vi "Mask Image to ROIs.vi"(8 "Error In":errorcluster, 9 "Max number of vectors in ROI (2500)":i32=2500, 10 "External edges only (T)":bool=TRUE, 11 "Mask Image Refnum in":T2) -> (0 "Error Out":errorcluster, 2 "ROIs":T1[](array[typedef]) {"Contours"."Type" items=["No Selection", "Point", "Line", "Rectangle", "Oval", "Polygon", "Freehand Region", "Annulus", "Unused2", "Unused3", "Broken Line", "Freehand Line", "Rotated Rectangle"]}, 3 "Mask Image Refnum out":T2)   [LabVIEW 2021, in "Image.lvlib"]
uses:
  <vilib>/vision/Image Controls.llb/IMAQ Image.ctl
  <userlib>/_OpenG.lib/array/array.llb/Filter 1D Array with Scalar (I32)__ogtk.vi
  Image.lvlib
  <vilib>/vision/NI_Vision_Development_Module.lvlib
  <userlib>/_OpenG.lib/array/array.llb/openg_array.lvlib
panel:
  out "# ROIs":i32
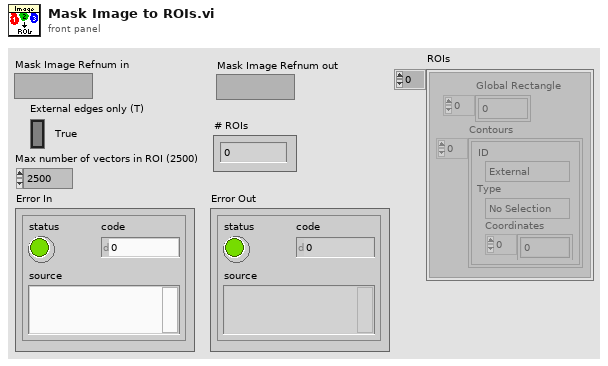
[diagram p1: front panel]
types:
  T1 = typedef "ROI Descriptor" = cluster{"Global Rectangle":i32[], "Contours":cluster{"ID":enum32{"External", "Internal"}, "Type":u32, "Coordinates":i32[]}[]}
  T2 = typedef "IMAQ Image.ctl" = refnum<image>
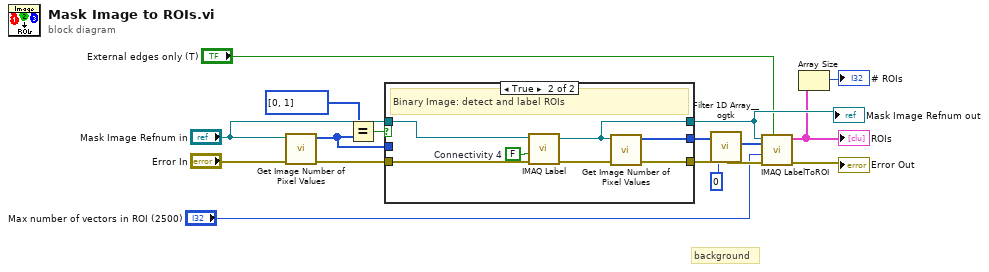
[diagram p0: block diagram]
diagram:
  # "background"
  n1 = call "Get Image Number of Pixel Values.vi"("Error In"="Error In", "Image"="Mask Image Refnum in") -> ("Error Out"=w5:errorcluster, "Pixel Values"=w4:i32[])  [unwired: 7 in, 1 out]
  n2 = Equal?(x=i32[] [0, 1] ("Pixel Values"), y=w4) -> (x = y?=w6:bool)
  n3 = case shown="True" w6 {
    tunnel: w5 -> [w19 w26]
    tunnel: [w19 w22] -> w16
    tunnel: w4 -> [w18 _]
    tunnel: [w18 w21] -> w3
    tunnel: "Mask Image Refnum in" -> [w17 w25]
    tunnel: [w17 w24] -> w15
    frame False {
      # "labeled image: next step"
    }
    frame True {
      w20 = FALSE  # Connectivity 4
      # "Binary Image: detect and label ROIs"
      n4 = call "IMAQ Label"("error in (no error)"=w26, "Connectivity 4/8 (8)"=w20, "Image Src"=w25) -> ("error out"=w23:errorcluster, "Image Dst Out"=w24:T2)  [unwired: 1 in, 1 out]
      n5 = call "Get Image Number of Pixel Values.vi"("Error In"=w23, "Image"=w24) -> ("Error Out"=w22:errorcluster, "Pixel Values"=w21:i32[])  [unwired: 7 in, 1 out]
    }
  }
  "Mask Image Refnum out" <- w15
  n6 = call-poly <userlib>:"Filter 1D Array__ogtk.vi"("items to filter"=0, "array"=w3) -> ("filtered array"=w2:i32[])  [unwired: 4 in, 1 out]
  n7 = call "IMAQ LabelToROI"("External edges only (T)"="External edges only (T)", "error in (no error)"=w16, "Max number of vectors in ROI"="Max number of vectors in ROI (2500)", "Labels In"=w2, "Image"=w15) -> ("error out"=→"Error Out":errorcluster, "ROIs"=w9:T1[])  [unwired: 3 in, 2 out]
  "ROIs" <- w9
  n8 = Array Size(array=w9) -> (size(s)=→"# ROIs":i32)
